vi "getName.vi"(8 "error in (no error)":errorcluster, 11 "AbstractCustomer in":refnum<class "AbstractCustomer.lvclass">) -> (0 "error out":errorcluster, 2 "name":string, 3 "AbstractCustomer out":refnum<class "AbstractCustomer.lvclass">)   [LabVIEW 2017, in "AbstractCustomer.lvclass"]
uses:
  AbstractCustomer.lvclass
  AbstractCustomer.lvclass/AbstractCustomer.ctl
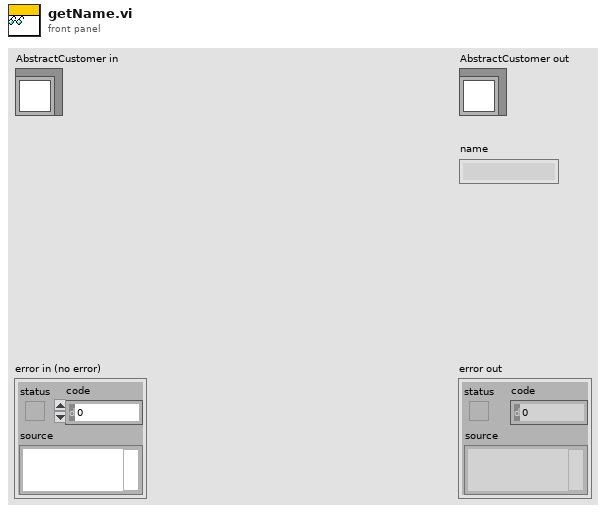
[diagram p1: front panel]
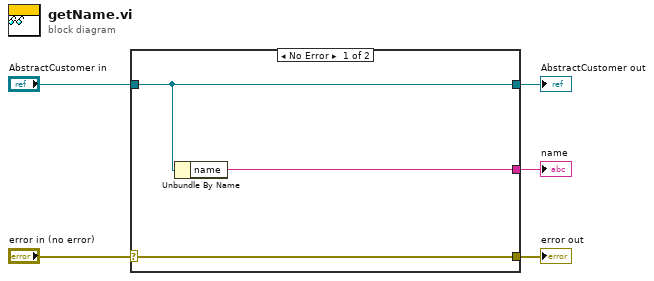
[diagram p0: block diagram]
diagram:
  n1 = case shown="No Error" "error in (no error)" {
    selector: "error in (no error)" -> [w8 w9]
    tunnel: [w8 w9] -> w4
    tunnel: [w7 w10] -> w2
    tunnel: "AbstractCustomer in" -> [w7 w10]
    tunnel: [w6 _] -> w1
    frame No Error {
      n2 = Unbundle By Name(w7) -> ("name"=w6:string)
    }
    frame Error {
    }
  }
  "error out" <- w4
  "AbstractCustomer out" <- w2
  "name" <- w1
